vi "Temperature Limit.vi"() -> ()   [LabVIEW 2012]
doc: "该VI可仿真温度采集，绘制温度图形，并通知用户温度是否超出范围。"
panel:
  in  "开始":bool
  in  "△t(ms)":i32(slide)=400 scale=50.0..500.0
  in  "停止":bool
  in  "上限":dbl=28.0 format="%.2f"
  out "温度":cluster{"Temperature":dbl, "High Limit":dbl}(graph)={"Temperature"=85.88749999999999, "High Limit"=80.0}
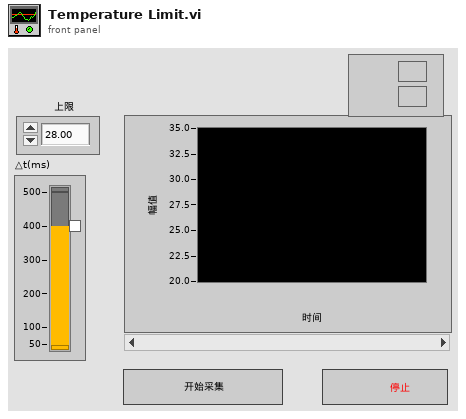
[diagram p1: front panel]
types:
  T1 = enum8{"Enabled", "Disabled", "Disabled and Grayed Out"}
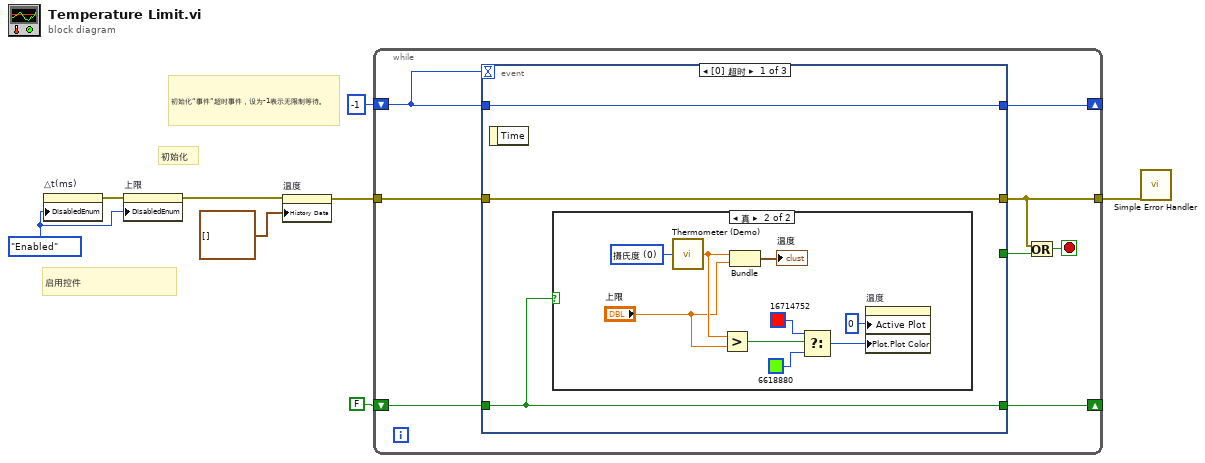
[diagram p0: block diagram]
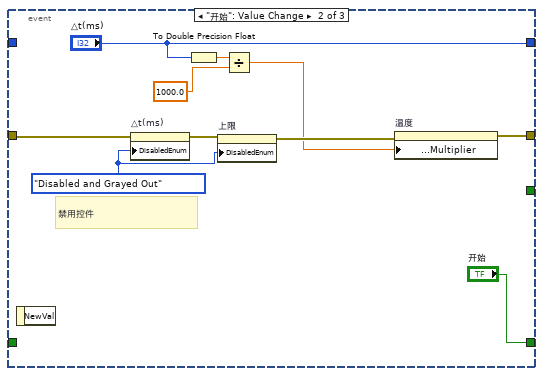
[diagram p3: hidden frame]
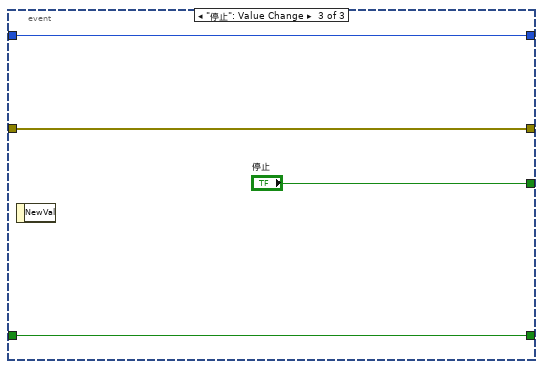
[diagram p4: hidden frame]
diagram:
  w6 = T1."Enabled" ("禁用")
  # "初始化“事件”超时事件，设为-1表示无限制等待。"
  # "启用控件"
  # "初始化"
  n1 = property on="△t(ms)" class="Slide (严格)"("DisabledEnum"=w6) -> (error out=w5:errorcluster)  [unwired: 2 in, 1 out]
  n2 = property on="上限" class="DigNum (严格)"(error in=w5, "DisabledEnum"=w6) -> (error out=w4:errorcluster)  [unwired: 1 in, 1 out]
  n3 = property on="温度" class="WFChart (严格)"(error in=w4, "History Data"=cluster{"温度":dbl, "高限制":dbl}[] [] ("历史数据")) -> (error out=w7:errorcluster)  [unwired: 1 in, 1 out]
  n4 = while {
    tunnel: w7 -> [w16]
    tunnel: [w14] -> w2
    shift-right: [w12] -> _
    shift-left: FALSE ("开始") -> [w11]
    shift-right: [w10] -> _
    shift-left: -1 ("△t(ms)") -> [w9]
    stop <- w15 stop-if-true
    n5 = event shown="[0] 超时" {
      selector: _ -> [_ _ _]
      dyn-events: _ -> [_ _ _]
      timeout: w9 -> [_ _ _]
      tunnel: [_ _ "停止"] -> w13
      tunnel: w16 -> [w19 w36 w41]
      tunnel: [w19 w34 w41] -> w14
      tunnel: [w17 "开始" w40] -> w12
      tunnel: w11 -> [w17 _ w40]
      tunnel: [w18 "△t(ms)" w39] -> w10
      tunnel: w9 -> [w18 _ w39]
      event Timeout {
        n6 = event-data ("事件数据节点")() -> ()  [unwired: 1 in, 1 out]
        n7 = case shown="真" w17 {
          frame False {
          }
          frame True {
            w20 = u16 0 items=["摄氏度", "华氏度"] ("单位（0：摄氏度）")
            n8 = call "Thermometer (Demo).vi"("单位（0：摄氏度）"=w20) -> ("温度值"=w27:dbl)
            n9 = Greater? ("大于？")(x=w27, y="上限") -> (0:w25:bool)
            n10 = Bundle ("捆绑")("温度值"=w27, "上限"="上限") -> (→"温度":cluster{"温度值":dbl, "上限":dbl})  [unwired: 1 in]
            n11 = Select ("选择")(t=u32 16714752, s=w25, f=u32 6618880) -> (s? t:f=w24:u32)
            n12 = property on="温度" class="WFChart (严格)"("Active Plot"=u32 0 ("活动曲线"), "Plot.Plot Color"=w24) -> ()  [unwired: 2 in, 2 out]
          }
        }
      }
      event "开始": Value Change {
        w37 = T1."Disabled and Grayed Out" ("禁用")
        # "禁用控件"
        n13 = event-data ("事件数据节点")() -> ()  [unwired: 1 in, 1 out]
        n14 = property on="△t(ms)" class="Slide (严格)"(error in=w36, "DisabledEnum"=w37) -> (error out=w38:errorcluster)  [unwired: 1 in, 1 out]
        n15 = To Double Precision Float ("转换为双精度浮点数")(number="△t(ms)") -> (double precision float=w33:dbl)
        n16 = property on="上限" class="DigNum (严格)"(error in=w38, "DisabledEnum"=w37) -> (error out=w35:errorcluster)  [unwired: 1 in, 1 out]
        n17 = Divide ("除")(x=w33, y=1000.0) -> (x/y=w31:dbl)
        n18 = property on="温度" class="WFChart (严格)"(error in=w35, "X Scale.Offset and Multiplier:Multiplier"=w31) -> (error out=w34:errorcluster)  [unwired: 1 in, 1 out]
      }
      event "停止": Value Change {
        n19 = event-data ("事件数据节点")() -> ()  [unwired: 1 in, 1 out]
      }
    }
    n20 = Or ("或")(x=w14, y=w13) -> (x .or. y?=w15:bool)
  }
  n21 = call <vilib>:"Simple Error Handler.vi"("error in (no error)"=w2) -> ()  [unwired: 4 in, 5 out]
